vi "MAIN.vi"() -> ()   [LabVIEW 2024]
uses:
  Program Files/National Instruments/LabVIEW 2024/examples/Instrument IO/Serial/support/Serial - Settings.ctl
  <vilib>/Instr/_visa.llb/VISA Configure Serial Port (Instr).vi
panel:
  out "error out":errorcluster
  out "Actual State":T1(ring)
  out "Next state":T1(ring)
  in  "Number of samples":i32 min=1 max=20
  in  "Serial Settings":T2={"baud rate"=9600, "data bits"=8, "parity"=enum."None", "stop bits"=10, "flow control"=0} {"flow control" items=["None"=0, "XON/XOFF"=1, "RTS/CTS"=2, "DTR/DSR"=4]; "stop bits" items=["1.0"=10, "1.5"=15, "2.0"=20]; "data bits" min=5 max=8 step=1; "baud rate" items=["75"=75, "110"=110, "134"=134, "150"=150, "300"=300, "600"=600, "1200"=1200, "1800"=1800, "2400"=2400, "4800"=4800, "7200"=7200, "9600"=9600, "14400"=14400, "19200"=19200, "28800"=28800, "38400"=38400, "56000"=56000, "57600"=57600, "115200"=115200, "128000"=128000, "230400"=230400]}
  out "bytes read":u32
  out "Response":string
  in  "delay before read (ms)":u32=500
  in  "VISA resource name":refnum<visa-resource-name>="COM1"
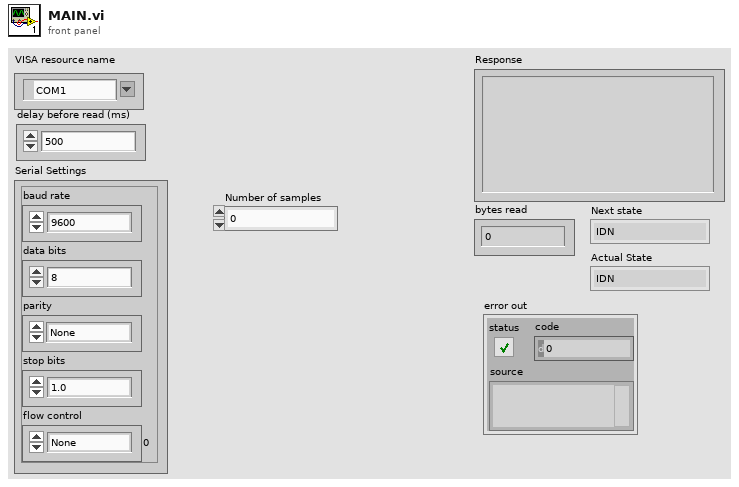
[diagram p1: front panel]
types:
  T1 = enum16{"IDN", "REMOTE_SET", "MEAS_SET", "AVERAGE", "DONE"}
  T2 = typedef "Serial - Settings.ctl" = cluster{"baud rate":u32, "data bits":u16, "parity":enum16{"None", "Odd", "Even", "Mark", "Space"}, "stop bits":u16, "flow control":u16}
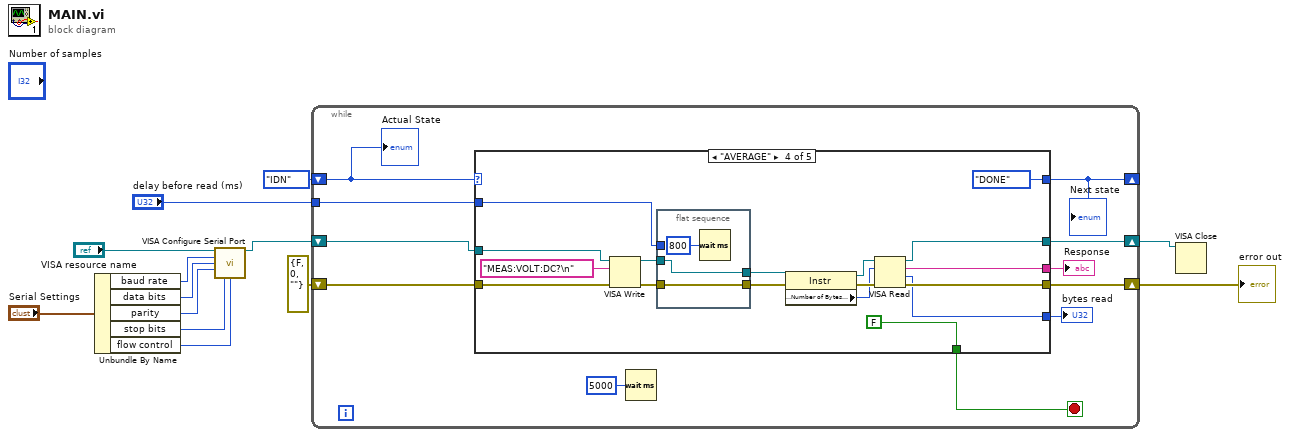
[diagram p0: block diagram]
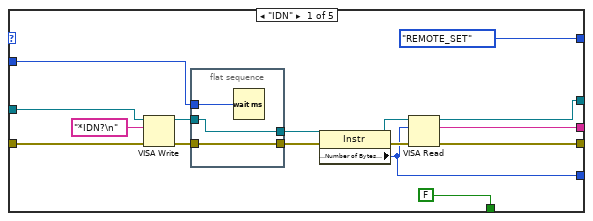
[diagram p2: hidden frame]
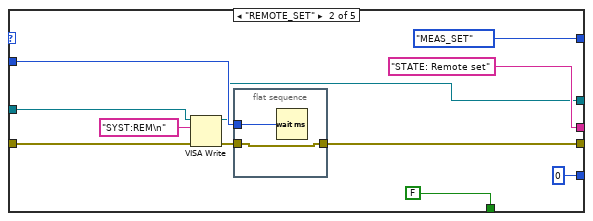
[diagram p3: hidden frame]
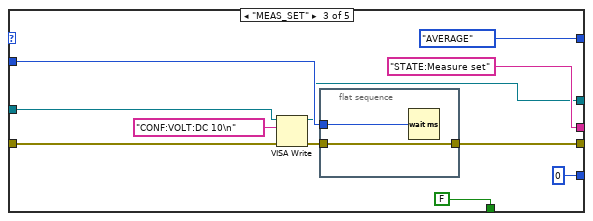
[diagram p4: hidden frame]
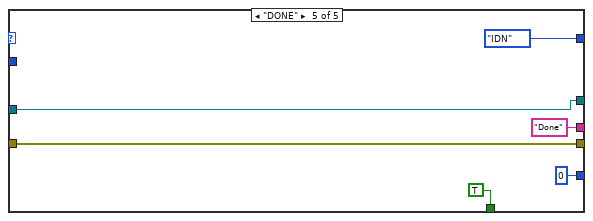
[diagram p5: hidden frame]
diagram:
  n1 = Unbundle By Name("Serial Settings") -> ("baud rate"=w11:u32, "data bits"=w9:u16, "parity"=w10:enum16{"None", "Odd", "Even", "Mark", "Space"}, "stop bits"=w8:u16, "flow control"=w7:u16)
  n2 = call-poly "VISA Configure Serial Port"("VISA resource name"="VISA resource name", "baud rate (9600)"=w11, "data bits (8)"=w9, "parity (0:none)"=w10, "stop bits (10: 1 bit)"=w8, "flow control (0:none)"=w7) -> ("VISA resource name out"=w6:refnum<visa-resource-name>)  [unwired: 3 in, 6 out]
  n3 = while {
    tunnel: "delay before read (ms)" -> [w23]
    shift-right: [w22] -> _
    shift-left: T1."IDN" -> [w16]
    shift-right: [w21] -> w2
    shift-left: errorcluster {"status"=FALSE, "code"=0, "source"=""} ("error out") -> [w20]
    shift-right: [w14] -> w1
    shift-left: w6 -> [w24]
    stop <- w19 stop-if-true
    n4 = case shown="\"AVERAGE\"" w16 {
      tunnel: w24 -> [w33 w51 w64 w78 w90]
      tunnel: w23 -> [w32 w52 w65 w77 _]
      tunnel: [w31 u32 0 ("Bytes at Port") u32 0 ("Bytes at Port") w73 u32 0 ("return count")] -> w15
      tunnel: [w30 "STATE: Remote set" ("read buffer") "STATE:Measure set" ("read buffer") w76 "Done" ("read buffer")] -> w17
      tunnel: [T1."REMOTE_SET" T1."MEAS_SET" T1."AVERAGE" T1."DONE" T1."IDN"] -> w22
      tunnel: [w27 w50 w62 w75 w95] -> w21
      tunnel: w20 -> [w28 w49 w63 w74 w95]
      tunnel: [FALSE FALSE FALSE FALSE TRUE] -> w19
      tunnel: [w25 w44 w57 w70 w90] -> w14
      frame "IDN" {
        n5 = VISA Write(VISA resource name=w33, write buffer="*IDN?\n" ("Command"), error in (no error)=w28) -> (VISA resource name out=w37:refnum<visa-resource-name>, error out=w35:errorcluster)  [unwired: 1 out]
        n6 = flat-sequence {
          tunnel: w35 -> [w43]
          tunnel: [w43] -> w36
          tunnel: w37 -> [w42]
          tunnel: [w42] -> w38
          tunnel: w32 -> [w41]
          frame #0 {
            n7 = Wait (ms)(milliseconds to wait=w41) -> ()  [unwired: 1 out]
          }
        }
        n8 = property class="Instr"(reference=w38, error in=w36) -> (reference out=w39:refnum<visa-resource-name>, error out=w40:errorcluster, "Serial Settings:Number of Bytes at Serial Port"=w31:u32)
        n9 = VISA Read(VISA resource name=w39, byte count=w31, error in (no error)=w40) -> (VISA resource name out=w25:refnum<visa-resource-name>, read buffer=w30:string, error out=w27:errorcluster)  [unwired: 1 out]
      }
      frame "REMOTE_SET" {
        n10 = VISA Write(VISA resource name=w51, write buffer="SYST:REM\n" ("Command"), error in (no error)=w49) -> (VISA resource name out=w44:refnum<visa-resource-name>, error out=w54:errorcluster)  [unwired: 1 out]
        n11 = flat-sequence {
          tunnel: w54 -> [w56]
          tunnel: [w56] -> w50
          tunnel: w52 -> [w55]
          frame #0 {
            n12 = Wait (ms)(milliseconds to wait=w55) -> ()  [unwired: 1 out]
          }
        }
      }
      frame "MEAS_SET" {
        n13 = VISA Write(VISA resource name=w64, write buffer="CONF:VOLT:DC 10\n" ("Command"), error in (no error)=w63) -> (VISA resource name out=w57:refnum<visa-resource-name>, error out=w67:errorcluster)  [unwired: 1 out]
        n14 = flat-sequence {
          tunnel: w67 -> [w69]
          tunnel: [w69] -> w62
          tunnel: w65 -> [w68]
          frame #0 {
            n15 = Wait (ms)(milliseconds to wait=w68) -> ()  [unwired: 1 out]
          }
        }
      }
      frame "AVERAGE" {
        n16 = VISA Write(VISA resource name=w78, write buffer="MEAS:VOLT:DC?\n" ("Command"), error in (no error)=w74) -> (VISA resource name out=w83:refnum<visa-resource-name>, error out=w81:errorcluster)  [unwired: 1 out]
        n17 = flat-sequence {
          tunnel: w81 -> [w89]
          tunnel: [w89] -> w82
          tunnel: w83 -> [w88]
          tunnel: [w88] -> w84
          tunnel: w77 -> [_]
          frame #0 {
            n18 = Wait (ms)(milliseconds to wait=u32 800) -> ()  [unwired: 1 out]
          }
        }
        n19 = property class="Instr"(reference=w84, error in=w82) -> (reference out=w85:refnum<visa-resource-name>, error out=w86:errorcluster, "Serial Settings:Number of Bytes at Serial Port"=w79:u32)
        n20 = VISA Read(VISA resource name=w85, byte count=w79, error in (no error)=w86) -> (VISA resource name out=w70:refnum<visa-resource-name>, read buffer=w76:string, return count=w73:u32, error out=w75:errorcluster)
      }
      frame "DONE" {
      }
    }
    "Response" <- w17
    "Next state" <- w22
    "bytes read" <- w15
    n21 = Wait (ms)(milliseconds to wait=u32 5000) -> ()  [unwired: 1 out]
    "Actual State" <- w16
  }
  "error out" <- w2
  n22 = VISA Close(VISA resource name=w1) -> ()  [unwired: 1 in, 1 out]
